vi "Main.vi"() -> ()   [LabVIEW 2017]
uses:
  Page-XControl/Page-XControl.xctl
  Slide/Slide.lvclass
panel:
  in  "Open":bool
  out "PageXCtrl":u32(xcontrol)
  in  "Stop":bool
  in  "Last":bool
  in  "First":bool
  in  "Left":bool
  in  "Right":bool
  out "LowerLeft":string caption="String"
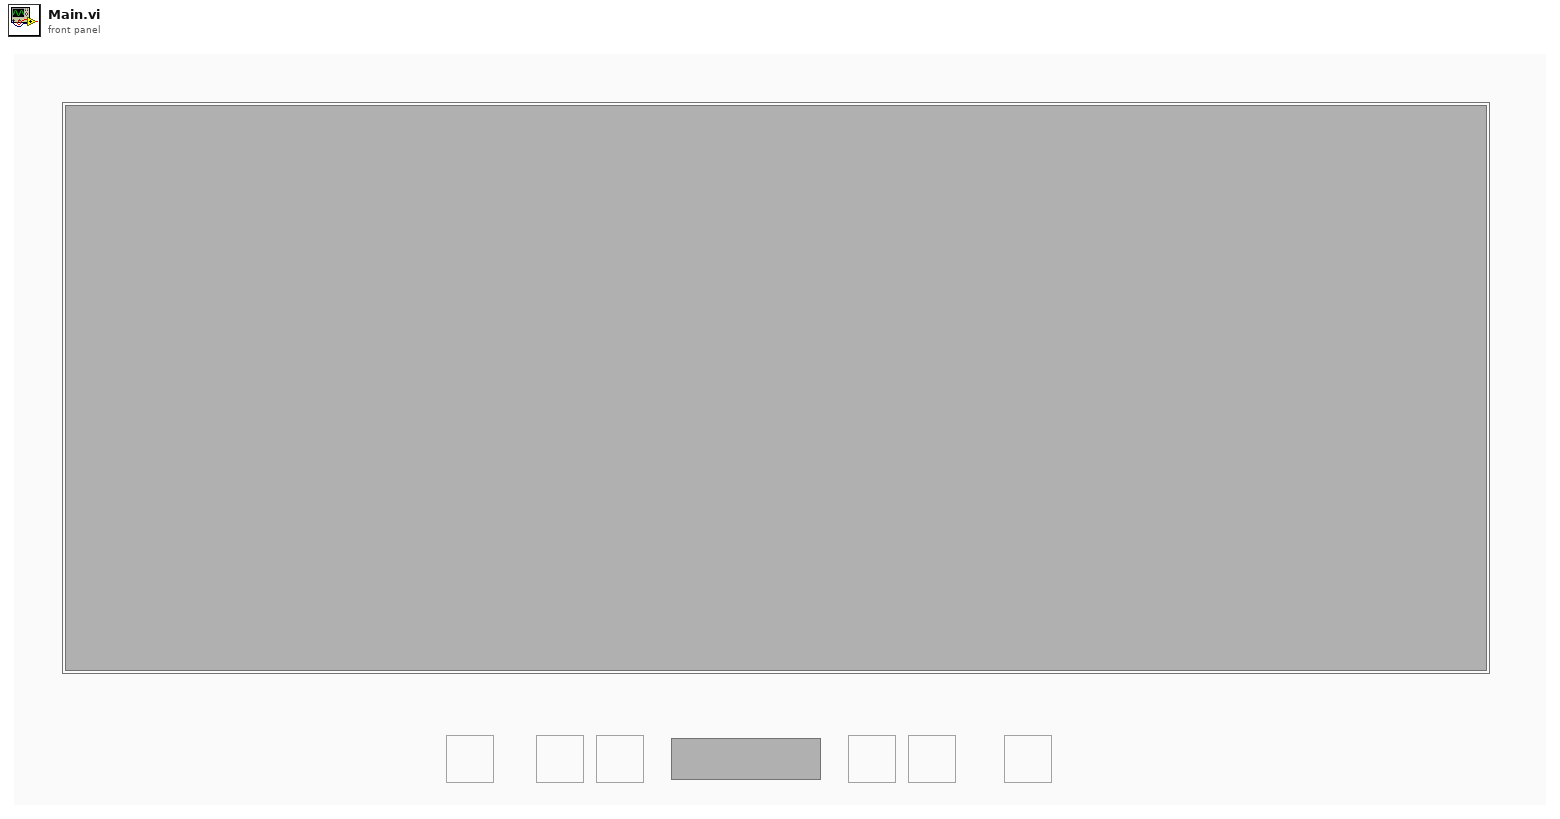
[diagram p1: front panel]
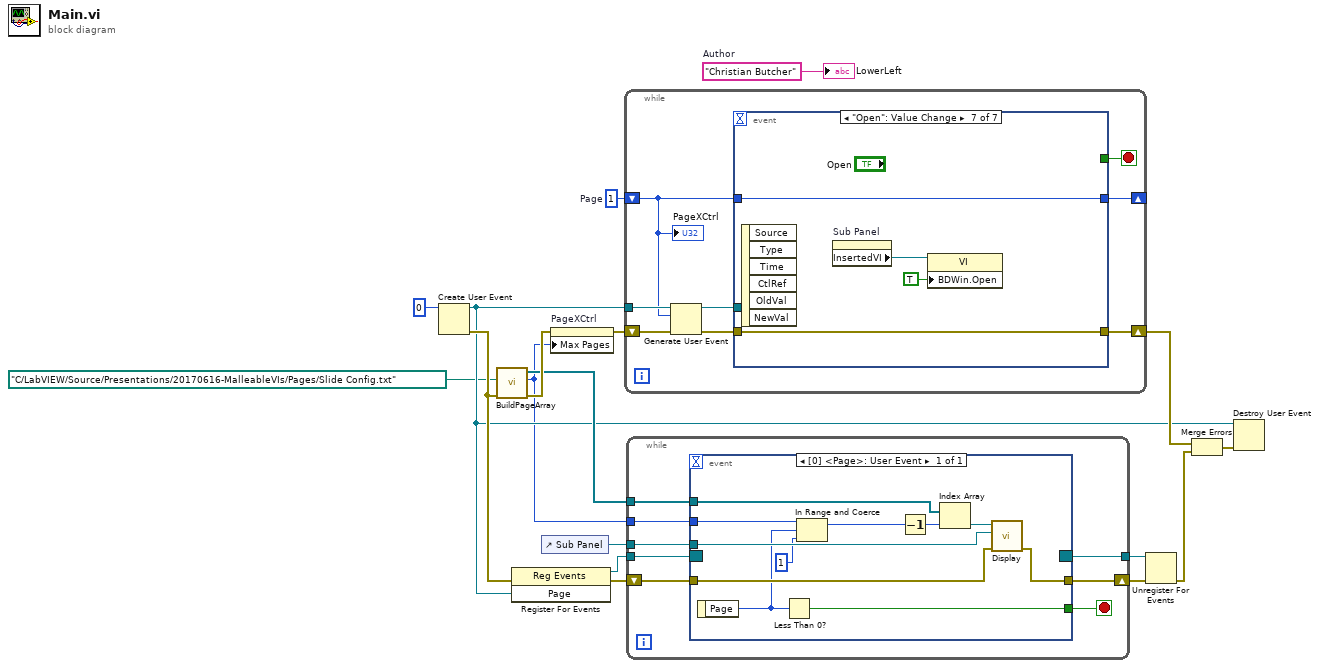
[diagram p0: block diagram]
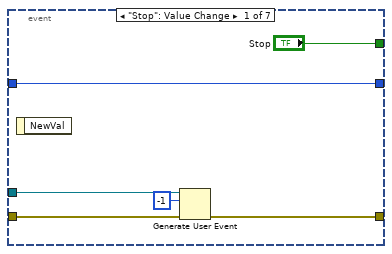
[diagram p2: hidden frame]
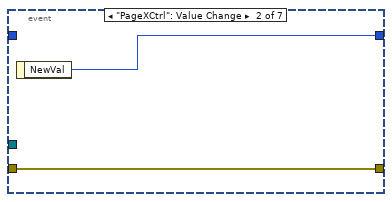
[diagram p3: hidden frame]
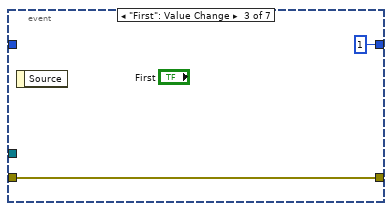
[diagram p4: hidden frame]
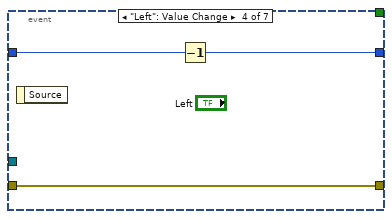
[diagram p5: hidden frame]
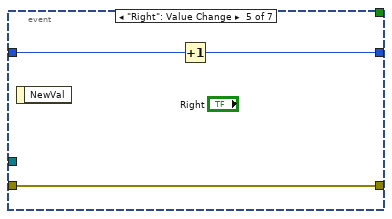
[diagram p6: hidden frame]
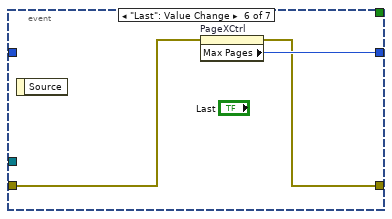
[diagram p7: hidden frame]
diagram:
  w16 = "Christian Butcher"  # Author
  w17 = u32 1  # Page
  n1 = Create User Event(user event datatype=0 ("Page")) -> (user event=w4:refnum<user-event>, error out=w13:errorcluster)  [unwired: 1 in]
  n2 = call "BuildPageArray.vi"("error in (no error)"=w13, "Config File Path"=path "C:/LabVIEW/Source/Presentations/20170616-MalleableVIs/Pages/Slide Config.txt") -> ("error out"=w18:errorcluster, "Num Pages"=w1:i32, "Array"=w10:refnum<class "Slide.lvclass">[])  [unwired: 7 in]
  n3 = register-events(error in=w13, w4) -> (reference out=w11:refnum<event-registration>, error out=w12:errorcluster)  [unwired: 1 in]
  n4 = control-ref of="Sub Panel"() -> (w2:refnum<vi>)
  n5 = property on="PageXCtrl" class="Page-XControl (strict)"(error in=w18, "Max Pages"=w1) -> (error out=w15:errorcluster)  [unwired: 1 in, 1 out]
  n6 = while {
    shift-right: [w25] -> _
    shift-left: w17 -> [w20]
    shift-right: [w23] -> w7
    shift-left: w15 -> [w24]
    tunnel: w4 -> [w21]
    stop <- w26 stop-if-true
    n7 = Generate User Event(user event=w21, event data cluster=w20, error in=w24) -> (user event out=w19:refnum<user-event>, error out=w22:errorcluster)  [unwired: 1 in]
    n8 = event shown="[6] \"Open\": Value Change" {
      selector: _ -> [_ _ _ _ _ _ _]
      dyn-events: _ -> [_ _ _ _ _ _ _]
      timeout: _ -> [_ _ _ _ _ _ _]
      tunnel: ["Stop" _ _ _ _ _ _] -> w26
      tunnel: w20 -> [w32 _ _ w39 w42 _ w49]
      tunnel: [w32 w33 u32 1 ("NewVal") w38 w41 w45 w49] -> w25
      tunnel: w22 -> [w30 w34 w36 w37 w40 w44 w48]
      tunnel: [w29 w34 w36 w37 w40 w43 w48] -> w23
      tunnel: w19 -> [w28 _ _ _ _ _ _]
      event "Stop": Value Change {
        n9 = event-data() -> ()  [unwired: 1 in, 1 out]
        n10 = Generate User Event(user event=w28, event data cluster=-1 ("event data"), error in=w30) -> (error out=w29:errorcluster)  [unwired: 1 in, 1 out]
      }
      event "PageXCtrl": Value Change {
        n11 = event-data() -> ("NewVal"=w33:u32)  [unwired: 1 in]
      }
      event "First": Value Change {
        n12 = event-data() -> ()  [unwired: 1 in, 1 out]
      }
      event "Left": Value Change {
        n13 = event-data() -> ()  [unwired: 1 in, 1 out]
        n14 = Decrement(x=w39) -> (x-1=w38:u32)
      }
      event "Right": Value Change {
        n15 = event-data() -> ()  [unwired: 1 in, 1 out]
        n16 = Increment(x=w42) -> (x+1=w41:u32)
      }
      event "Last": Value Change {
        n17 = event-data() -> ()  [unwired: 1 in, 1 out]
        n18 = property on="PageXCtrl" class="Page-XControl (strict)"(error in=w44) -> (error out=w43:errorcluster, "Max Pages"=w45:u32)  [unwired: 1 in, 1 out]
      }
      event "Open": Value Change {
        n19 = event-data() -> ()  [unwired: 1 in, 6 out]
        n20 = property on="Sub Panel" class="SubPnl"() -> ("InsertedVI"=w47:refnum<vi>)  [unwired: 2 in, 2 out]
        n21 = property on="Property Node" class="VI"(reference=w47, "BDWin.Open"=TRUE ("Block Diagram Window:Open")) -> ()  [unwired: 1 in, 2 out]
      }
    }
    "PageXCtrl" <- w20
  }
  n22 = while {
    tunnel: w11 -> [w56]
    shift-right: [w53] -> w9
    shift-left: w12 -> [w57]
    tunnel: w10 -> [w54]
    tunnel: [w52] -> w8
    tunnel: w2 -> [w51]
    tunnel: w1 -> [w50]
    stop <- w55 stop-if-true
    n23 = event shown="[0] <Page>: User Event" {
      selector: w56 -> [_]
      dyn-events: [_] -> w52
      timeout: _ -> [_]
      tunnel: w57 -> [w65]
      tunnel: [w68] -> w55
      tunnel: w54 -> [w67]
      tunnel: [w64] -> w53
      tunnel: w51 -> [w66]
      tunnel: w50 -> [w63]
      event User Event {
        n24 = event-data() -> ("Page"=w62:i32)  [unwired: 1 in]
        n25 = Less Than 0?(x=w62) -> (x < 0?=w68:bool)
        n26 = In Range and Coerce(upper limit=w63, x=w62, lower limit=u32 1) -> (coerced(x)=w61:u32)  [unwired: 1 out]
        n27 = Decrement(x=w61) -> (x-1=w58:u32)
        n28 = Index Array(array=w67, index=w58) -> (element=w59:refnum<class "Slide.lvclass">)
        n29 = call-dynamic "Display.vi"("error in (no error)"=w65, "SubPnl Refnum"=w66, "Slide in"=w59) -> ("error out"=w64:errorcluster)  [unwired: 7 in, 1 out]
      }
    }
  }
  n30 = Unregister For Events(event registration refnum=w8, error in=w9) -> (error out=w6:errorcluster)
  n31 = Merge Errors(w7, w6) -> (w5:errorcluster)
  n32 = Destroy User Event(user event=w4, error in=w5) -> ()  [unwired: 1 out]
  "LowerLeft" <- w16
